vi "VI Server_OpenClustersRefs.vi"(8 "error in (no error)":errorcluster, 11 "VI Server Cluster":T1) -> (0 "error out":errorcluster, 3 "VI Server Cluster.DUP":T1)   [LabVIEW 2020, in "VI Server Toolkit LV2013.lvlib"]
doc: "Generates the VI Server cluster for cluster and adds it into incoming VI Server Cluster. This way controls/indicators of the cluster can be accessed the same way as \"stand alone\" GUI objects."
uses:
  VI Server Toolkit LV2013.lvlib
  VI Server_TypeDefs/VI Server_RefsCluster.ctl
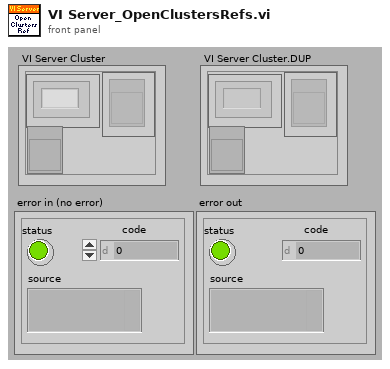
[diagram p1: front panel]
types:
  T1 = typedef "VI Server_RefsCluster.ctl" = cluster{"Labels":string[], "Refs":refnum<vi>[], "VI Ref":refnum<vi>}
  T2 = cluster{"ClassName":string, "CtrRef":refnum<vi>}[]
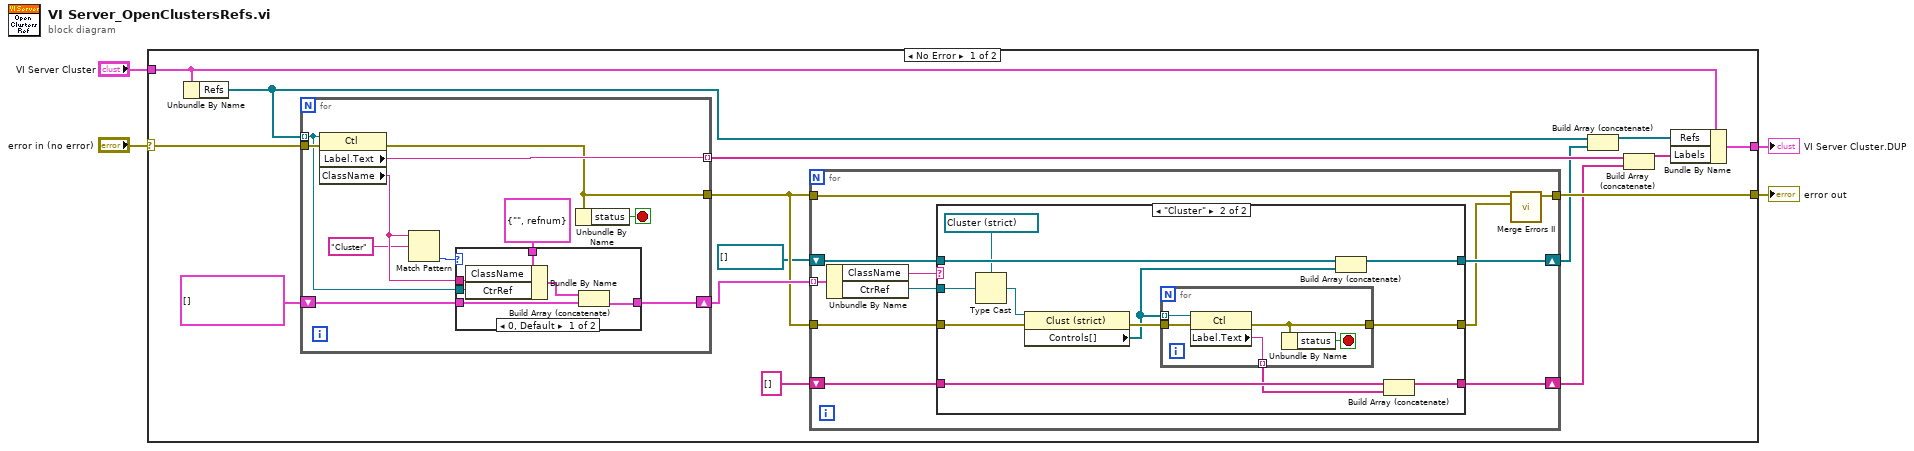
[diagram p0: block diagram]
diagram:
  n1 = case shown="No Error" "error in (no error)" {
    selector: "error in (no error)" -> [w5 w69]
    tunnel: [w15 w69] -> w4
    tunnel: [w19 _] -> w3
    tunnel: "VI Server Cluster" -> [w6 _]
    frame No Error {
      n2 = Unbundle By Name(w6) -> ("Refs"=w7:refnum<vi>[])
      n3 = for {
        tunnel: w7 -> [w56] mode=indexing
        tunnel: w5 -> [w61]
        tunnel: [w55] -> w14
        tunnel: [w60] -> w18 mode=indexing
        shift-right: [w58] -> w16
        shift-left: T2 [] -> [w59]
        stop <- w54 stop-if-true
        n4 = property class="Ctl"(reference=w56, error in=w61) -> (error out=w55:errorcluster, "Label.Text"=w60:string, "ClassName"=w53:string)  [unwired: 1 out]
        n5 = Match Pattern(string=w53, regular expression="Cluster") -> (offset past match=w51:i32)  [unwired: 1 in, 3 out]
        n6 = case shown="0, Default" w51 {
          tunnel: w59 -> [w67 w68]
          tunnel: [w66 w68] -> w58
          tunnel: cluster{"ClassName":string, "CtrRef":refnum<vi>} {"ClassName"="", "CtrRef"=refnum} -> [w65 _]
          tunnel: w53 -> [w64 _]
          tunnel: w56 -> [w63 _]
          frame 0, Default {
            n7 = Bundle By Name(cluster=w65, "ClassName"=w64, "CtrRef"=w63) -> (w62:cluster{"ClassName":string, "CtrRef":refnum<vi>})
            n8 = Build Array (concatenate)(w62, w67) -> (w66:T2)
          }
          frame -1 {
          }
        }
        n9 = Unbundle By Name(w55) -> ("status"=w54:bool)
      }
      n10 = for {
        tunnel: w16 -> [w30] mode=indexing
        tunnel: w14 -> [w22]
        tunnel: [w21] -> w15
        tunnel: w14 -> [w27]
        shift-right: [w24] -> w10
        shift-left: refnum<vi>[] [] ("Controls on Page[]") -> [w26]
        shift-right: [w23] -> w8
        shift-left: string[] [] -> [w25]
        n11 = Unbundle By Name(w30) -> ("ClassName"=w29:string, "CtrRef"=w28:refnum<vi>)
        n12 = case shown="\"Cluster\"" w29 {
          tunnel: w28 -> [_ w45]
          tunnel: w27 -> [w32 w38]
          tunnel: w26 -> [w31 w44]
          tunnel: w25 -> [w33 w43]
          tunnel: [w31 w42] -> w24
          tunnel: [w32 w41] -> w20
          tunnel: [w33 w40] -> w23
          frame "False", Default {
          }
          frame "Cluster" {
            n13 = Type Cast(type=refnum<vi> refnum ("error out"), x=w45) -> (*(type *) &x=w34:refnum<vi>)
            n14 = property class="Clust (strict)"(reference=w34, error in=w38) -> (error out=w37:errorcluster, "Controls[]"=w36:refnum<vi>[])  [unwired: 1 out]
            n15 = for {
              tunnel: w36 -> [w49] mode=indexing
              tunnel: w37 -> [w50]
              tunnel: [w48] -> w41
              tunnel: [w46] -> w35 mode=indexing
              stop <- w47 stop-if-true
              n16 = property class="Ctl"(reference=w49, error in=w50) -> (error out=w48:errorcluster, "Label.Text"=w46:string)  [unwired: 1 out]
              n17 = Unbundle By Name(w48) -> ("status"=w47:bool)
            }
            n18 = Build Array (concatenate)(w44, w36) -> (w42:refnum<vi>[])
            n19 = Build Array (concatenate)(w43, w35) -> (w40:string[])
          }
        }
        n20 = call "Merge Errors II.vi"("error in 2 (no error)"=w20, "error in 1 (no error)"=w22) -> ("error out.DUP"=w21:errorcluster)  [unwired: 4 in, 1 out]
      }
      n21 = Build Array (concatenate)(w7, w10) -> (w11:refnum<vi>[])
      n22 = Build Array (concatenate)(w18, w8) -> (w9:string[])
      n23 = Bundle By Name(cluster=w6, "Refs"=w11, "Labels"=w9) -> (w19:T1)
    }
    frame Error {
    }
  }
  "error out" <- w4
  "VI Server Cluster.DUP" <- w3
